vi "消息推送core.vi"(8 "error in (no error)":errorcluster caption="错误输入（无错误）", 10 "数组":string[](array[string])=["UID_u2gUaG5SHjMBZfWcukaJD0Ypef0K"], 11 "content":string) -> (0 "error out":errorcluster caption="错误输出", 3 "GBK":string)   [LabVIEW 2016, in "wxpusher.lvlib"]
uses:
  wxpusher.lvlib
  <vilib>/httpClient/POSTBuffer.vi
  <vilib>/httpClient/LabVIEWHTTPClient.lvlib
panel:
  out "JSON字符串":string
  out "headers":string caption="头部"
  out "body":string caption="体部"
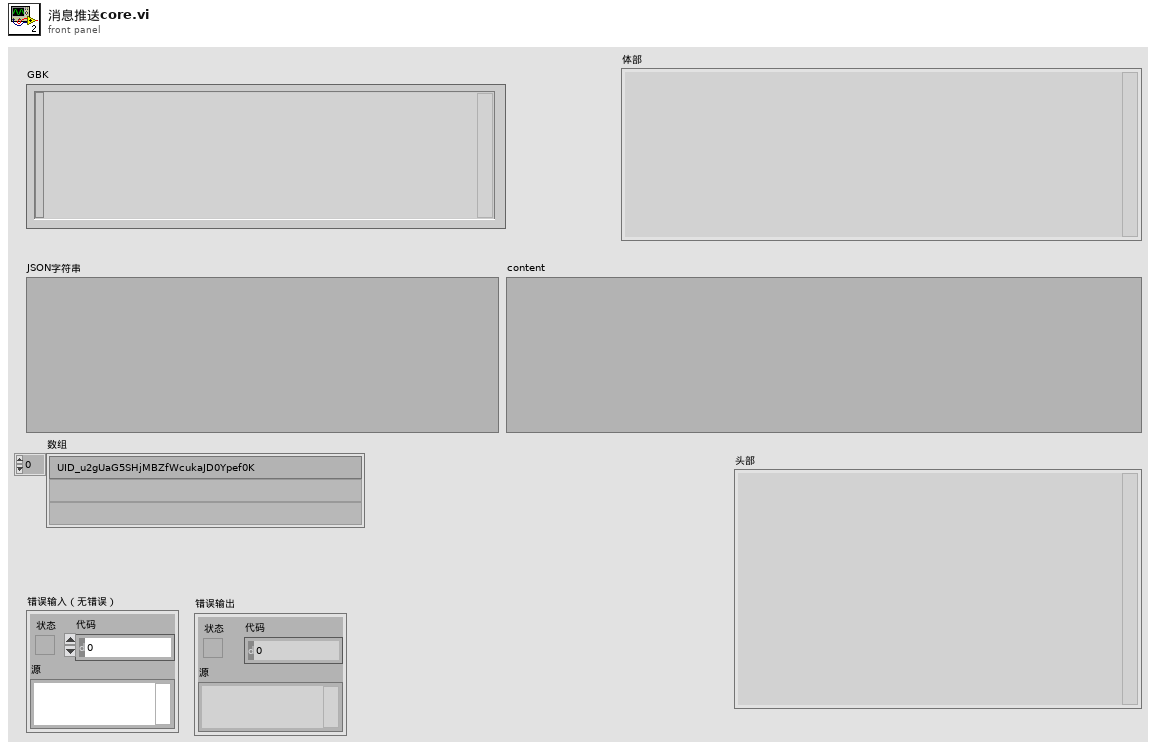
[diagram p1: front panel]
types:
  T1 = cluster{"appToken":string, "content":string, "contentType":i32, "topicIds":i32[], "uids":string[], "url":string}
  T2 = typedef "LabVIEWHTTPClient.lvlib/ClientHandle.ctl" = refnum<k1>
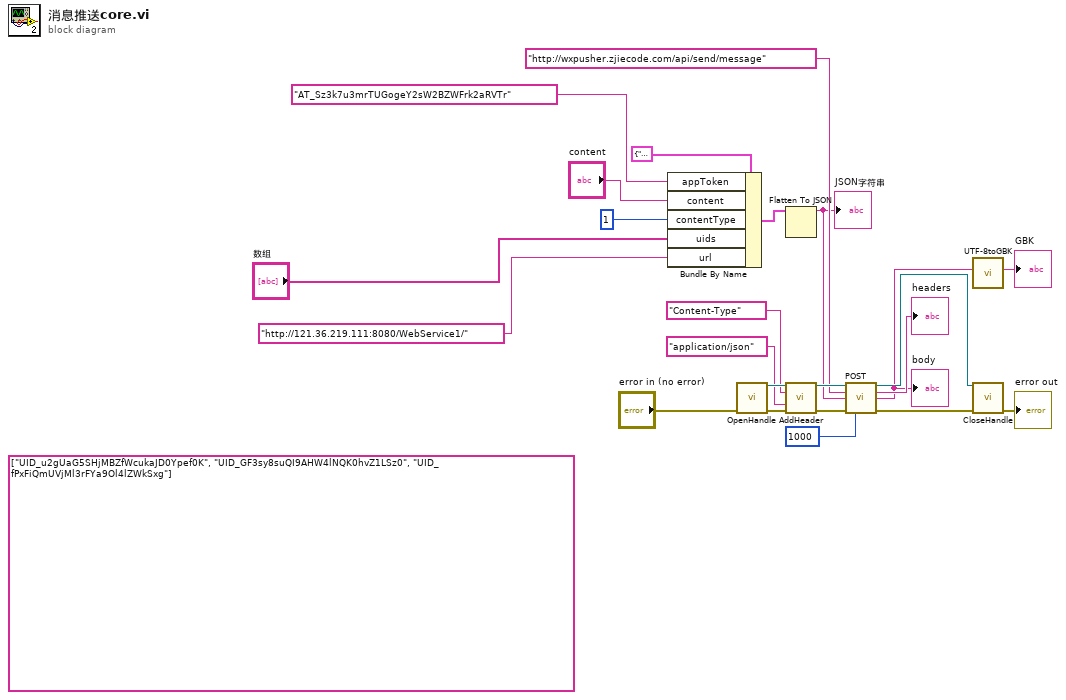
[diagram p0: block diagram]
diagram:
  (unwired) string[] ["UID_u2gUaG5SHjMBZfWcukaJD0Ypef0K", "UID_GF3sy8suQI9AHW4lNQK0hvZ1LSz0", "UID_fPxFiQmUVjMl3rFYa9Ol4lZWkSxg"]
  n1 = Bundle By Name(cluster=T1 {"appToken"="", "content"="", "contentType"=0, "topicIds"=[], "uids"=[], "url"=""}, "appToken"="AT_Sz3k7u3mrTUGogeY2sW2BZWFrk2aRVTr", "content"="content", "contentType"=1, "uids"="数组", "url"="http://121.36.219.111:8080/WebService1/" ("输入 5")) -> (w10:T1)
  n2 = call <vilib>:"OpenHandle.vi"("error in (no error)"="error in (no error)") -> ("client handle out"=w23:T2, "error out"=w21:errorcluster)  [unwired: 13 in]
  n3 = Flatten To JSON(anything=w10) -> (JSON string=w9:string)  [unwired: 2 in, 1 out]
  "JSON字符串" <- w9
  n4 = call <vilib>:"AddHeader.vi"("client handle"=w23, "header"="Content-Type", "value"="application/json", "error in (no error)"=w21) -> ("client handle out"=w22:T2, "error out"=w18:errorcluster)  [unwired: 10 in]
  n5 = call-poly <vilib>:"POST.vi"("client handle"=w22, "url"="http://wxpusher.zjiecode.com/api/send/message", "buffer"=w9, "error in (no error)"=w18, "timeout (10000)"=1000) -> ("client handle out"=w15:T2, "headers"=→"headers":string, "body"=w8:string, "error out"=w16:errorcluster)  [unwired: 7 in]
  "body" <- w8
  n6 = call "UTF-8toGBK.vi"("UTF-8"=w8) -> ("GBK"=→"GBK":string)  [unwired: 9 in, 1 out]
  n7 = call <vilib>:"CloseHandle.vi"("client handle"=w15, "error in (no error)"=w16) -> ("error out"=→"error out":errorcluster)  [unwired: 13 in]
